vi "Thev-Optimize Equivalent Source.vi"(0 "Frequency (Hz)":dbl[](array[numeric]), 5 "Px":cdb[][](array[numeric]), 9 "Options":T1, 11 "error in (no error)":errorcluster) -> (4 "Ps":cdb[](array[numeric]), 6 "Zs":cdb[](array[numeric]), 10 "Result":T2, 15 "error out":errorcluster)   [LabVIEW 2015]
uses:
  Typedefs/Thev-Optimization Result.ctl
  Typedefs/Thev-Optimization Parameters.ctl
  Utility VIs/Array Manipulation VIs/Irregular Array Subset (2D CDB).vi
  Utility VIs/Array Manipulation VIs/Irregular Array Subset (DBL).vi
  <vilib>/gmath/NumericalOptimization/Nonlinear Curve Fit LM.vi
  <vilib>/gmath/NI_Gmath.lvlib
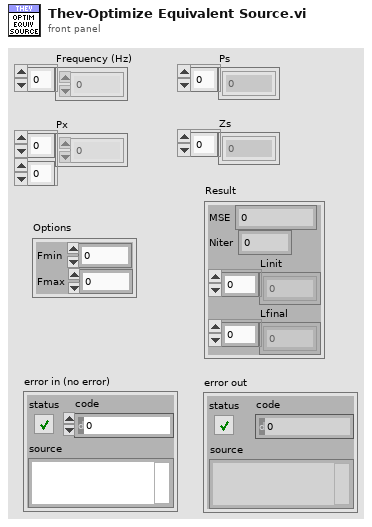
[diagram p1: front panel]
types:
  T1 = typedef "Thev-Optimization Parameters.ctl" = cluster{"Fmin":dbl, "Fmax":dbl}
  T2 = typedef "Thev-Optimization Result.ctl" = cluster{"MSE":dbl, "Niter":i32, "Linit":dbl[], "Lfinal":dbl[]}
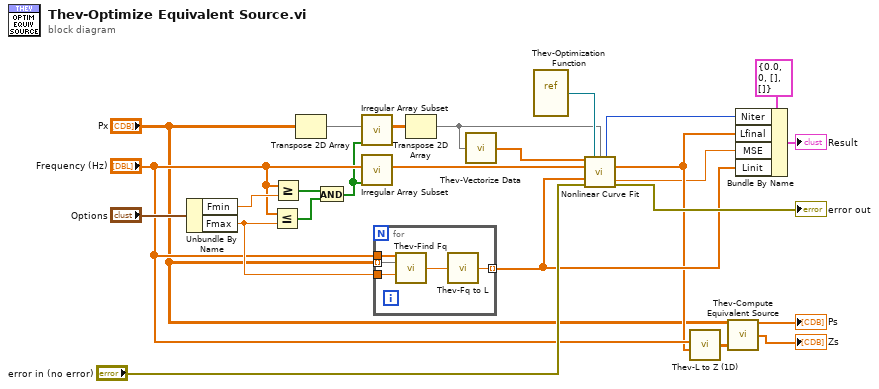
[diagram p0: block diagram]
diagram:
  n1 = Unbundle By Name("Options") -> ("Fmin"=w23:dbl, "Fmax"=w22:dbl)
  n2 = Less Or Equal?(x="Frequency (Hz)", y=w22) -> (x <= y?=w4:bool[])
  n3 = Greater Or Equal?(x="Frequency (Hz)", y=w23) -> (x >= y?=w24:bool[])
  n4 = Transpose 2D Array(2D array="Px") -> (transposed array=w16:cdb[][])
  n5 = And(x=w24, y=w4) -> (x .and. y?=w2:bool[])
  n6 = call-poly "Irregular Array Subset.vi"("Mask"=w2, "Array"=w16) -> ("Array Subset"=w19:cdb[][])  [unwired: 8 in, 1 out]
  n7 = call-poly "Irregular Array Subset.vi"("Mask"=w2, "Array"="Frequency (Hz)") -> ("Array Subset"=w21:dbl[])  [unwired: 8 in, 1 out]
  n8 = for {
    tunnel: "Px" -> [w29] mode=indexing
    tunnel: "Frequency (Hz)" -> [w28]
    tunnel: w22 -> [w27]
    tunnel: [w26] -> w12 mode=indexing
    n9 = call "Thev-Find Fq.vi"("Frequency (Hz)"=w28, "Px"=w29, "Fmax"=w27) -> ("Fq (Hz)"=w30:dbl)  [unwired: 12 in]
    n10 = call "Thev-Fq to L.vi"("Fq (Hz)"=w30) -> ("L (mm)"=w26:dbl)
  }
  n11 = Transpose 2D Array(2D array=w19) -> (transposed array=w15:cdb[][])
  n12 = call "Thev-Vectorize Data.vi"("2D CDB"=w15) -> ("1D DBL"=w3:dbl[])  [unwired: 14 in]
  n13 = vi-ref "Thev-Optimization Function.vi"() -> (w20:refnum<vi>)
  n14 = call-poly <vilib>:"Nonlinear Curve Fit.vi"("Y"=w3, "f(x,a)"=w20, "data"=w15, "X"=w21, "initial parameters"=w12, "error in (no error)"="error in (no error)") -> ("number of function calls"=w13:i32, "best fit parameters"=w9:dbl[], "residue"=w1:dbl, "error out"=→"error out":errorcluster)  [unwired: 4 in, 2 out]
  n15 = call "Thev-L to Z (1D).vi"("L (mm)"=w9, "Frequency (Hz)"="Frequency (Hz)") -> ("Zx"=w6:cdb[][])  [unwired: 2 in]
  n16 = call "Thev-Compute Equivalent Source.vi"("Px"="Px", "Zx"=w6) -> ("Ps"=→"Ps":cdb[], "Zs"=→"Zs":cdb[])  [unwired: 12 in]
  n17 = Bundle By Name(cluster=T2 {"MSE"=0.0, "Niter"=0, "Linit"=[], "Lfinal"=[]} ("Result"), "Niter"=w13, "Lfinal"=w9, "MSE"=w1, "Linit"=w12) -> (→"Result":T2)
